vi "FTW-Panel-FrontPanel-Open.vi"(6 "Bring to Front?":bool=TRUE, 8 "error in":errorcluster, 9 "Activate?":bool=TRUE, 10 "State":T1(ring)=enum."Standard", 11 "VI Ref":refnum<vi>) -> (0 "error out":errorcluster, 3 "VI Ref out":refnum<vi>)   [LabVIEW 2015]
panel:
  # "Inputs"
  # "Outputs"
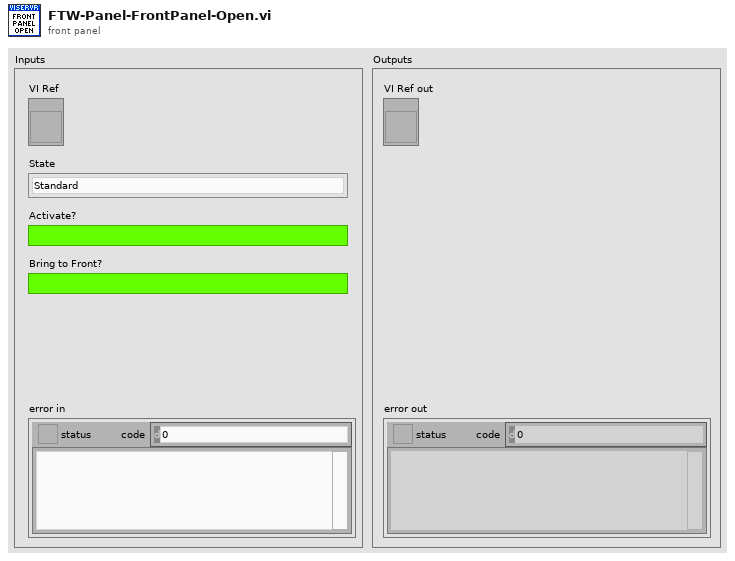
[diagram p1: front panel]
types:
  T1 = enum32{"Invalid", "Standard", "Closed", "Hidden", "Minimized", "Maximized"}
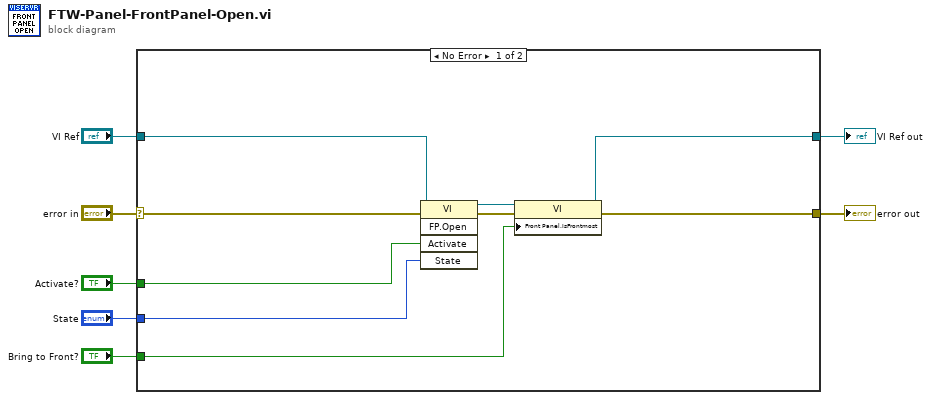
[diagram p0: block diagram]
diagram:
  n1 = case shown="No Error" "error in" {
    selector: "error in" -> [w16 w18]
    tunnel: [w10 w18] -> w7
    tunnel: "VI Ref" -> [w15 w17]
    tunnel: [w9 w17] -> w4
    tunnel: "Activate?" -> [w14 _]
    tunnel: "State" -> [w13 _]
    tunnel: "Bring to Front?" -> [w8 _]
    frame No Error {
      n2 = invoke class="VI" method="FP.Open"(reference=w15, error in=w16, "Activate"=w14, "State"=w13) -> (reference out=w12:refnum<vi>, error out=w11:errorcluster)  [unwired: 1 in, 3 out]
      n3 = property class="VI"(reference=w12, error in=w11, "Front Panel.IsFrontmost"=w8) -> (reference out=w9:refnum<vi>, error out=w10:errorcluster)
    }
    frame Error {
    }
  }
  "error out" <- w7
  "VI Ref out" <- w4
